vi "AES-InvCipher-text.vi"(5 "Initializer Vector":string, 7 "Operation Mode":T1, 8 "error in (no error)":errorcluster, 9 "inv-cipher [U8]":u8[](array[numeric]), 10 "Cipher Key":string, 11 "ciphertext":string) -> (0 "error out":errorcluster, 1 "inv-cipher out":u8[](array[numeric]), 3 "plaintext":string)   [LabVIEW 2020, in "Encryption.lvlib"]
doc: "Decipher a AES-encrypted message using the Cipher key and Operation Mode.\n\nCAUTION:\nThis VI is not secure, it does not protect the memory of the encryption, key and unencrypted data.\n\n(c) Ton Plomp, 2011\nTHIS SOFTWARE IS PROVIDED AS IS, AND ANY WARRANTY IS REJECTED"
uses:
  Encryption.lvlib
  AES-Modes.ctl
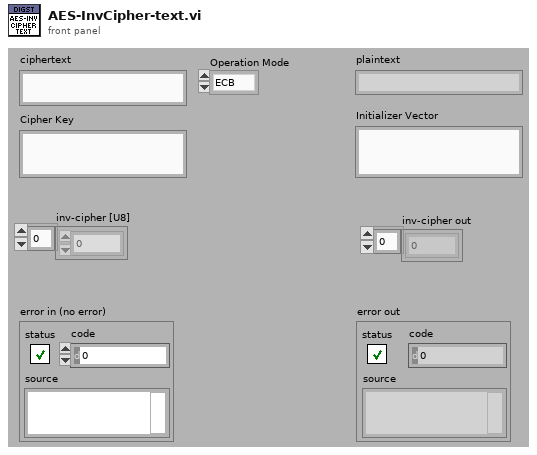
[diagram p1: front panel]
types:
  T1 = typedef "Encryption.lvlib/AES-Modes.ctl" = enum16{"ECB", "CBC", "CFB128", "OFB"}
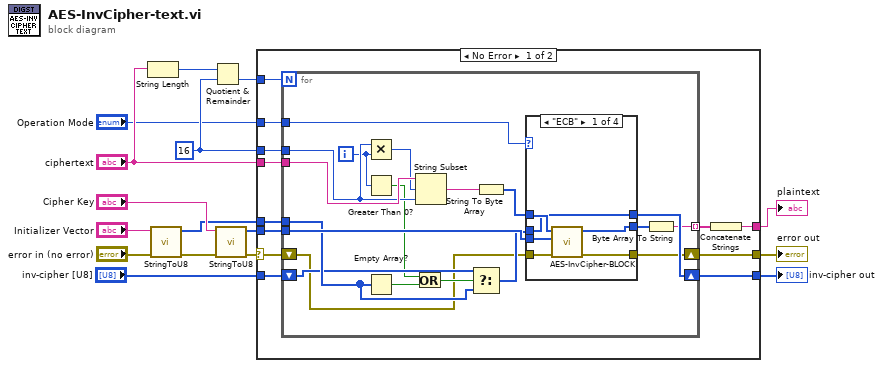
[diagram p0: block diagram]
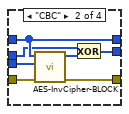
[diagram p2: hidden frame]
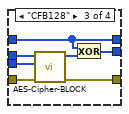
[diagram p3: hidden frame]
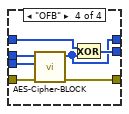
[diagram p4: hidden frame]
diagram:
  w9 = 16 ("y")
  n1 = String Length(string="ciphertext") -> (length=w13:i32)
  n2 = call "StringToU8.vi"("error in (no error)"="error in (no error)", "HEX text in"="Initializer Vector") -> ("error out"=w6:errorcluster, "ArrayU8 out"=w4:u8[])  [unwired: 8 in]
  n3 = Quotient & Remainder(x=w13, y=w9) -> (floor(x/y)=w8:i32)  [unwired: 1 out]
  n4 = call "StringToU8.vi"("error in (no error)"=w6, "HEX text in"="Cipher Key") -> ("error out"=w12:errorcluster, "ArrayU8 out"=w11:u8[])  [unwired: 8 in]
  n5 = case shown="No Error" w12 {
    selector: w12 -> [w24 w76]
    tunnel: "ciphertext" -> [w28 _]
    tunnel: [w23 w76] -> w15
    tunnel: w11 -> [w27 _]
    tunnel: w8 -> [w26 _]
    tunnel: w9 -> [w25 _]
    tunnel: [w21 _] -> w10
    tunnel: w4 -> [w19 _]
    tunnel: "Operation Mode" -> [w20 _]
    tunnel: "inv-cipher [U8]" -> [w18 w75]
    tunnel: [w17 w75] -> w1
    frame No Error {
      n6 = for {
        N: w26 -> [_]
        tunnel: w28 -> [w46]
        tunnel: w27 -> [w47]
        tunnel: w25 -> [w44]
        shift-right: [w39] -> w23
        shift-left: w24 -> [w31]
        tunnel: [w41] -> w22 mode=indexing
        shift-right: [w42] -> w17
        shift-left: w18 -> [w37]
        tunnel: w20 -> [w43]
        tunnel: w19 -> [w38]
        i -> [w35]
        n7 = Multiply(x=w44, y=w35) -> (x*y=w45:i32)
        n8 = Greater Than 0?(x=w35) -> (x > 0?=w34:bool)
        n9 = Empty Array?(array=w38) -> (empty?=w33:bool)
        n10 = Or(x=w34, y=w33) -> (x .or. y?=w32:bool)
        n11 = String Subset(string=w46, offset (0)=w45, length (rest)=w44) -> (substring=w30:string)
        n12 = Select(t=w37, s=w32, f=w38) -> (s? t:f=w36:u8[])
        n13 = String To Byte Array(string=w30) -> (unsigned byte array=w29:u8[])
        n14 = case shown="\"ECB\"" w43 {
          tunnel: w47 -> [w53 w60 w67 w74]
          tunnel: w29 -> [w52 w57 w61 w69]
          tunnel: w31 -> [w51 w59 w66 w73]
          tunnel: [w50 w54 w63 w71] -> w40
          tunnel: [w49 w58 w65 w72] -> w39
          tunnel: w36 -> [w48 w56 w62 w70]
          tunnel: [w48 w57 w61 w68] -> w42
          frame "ECB" {
            n15 = call "AES-InvCipher-BLOCK.vi"("error in (no error)"=w51, "Cipher Key"=w53, "cipher [U8]"=w52) -> ("error out"=w49:errorcluster, "plain [U8]"=w50:u8[])  [unwired: 7 in]
          }
          frame "CBC" {
            n16 = call "AES-InvCipher-BLOCK.vi"("error in (no error)"=w59, "Cipher Key"=w60, "cipher [U8]"=w57) -> ("error out"=w58:errorcluster, "plain [U8]"=w55:u8[])  [unwired: 7 in]
            n17 = Exclusive Or(1:w55, 2:w56) -> (0:w54:u8[])
          }
          frame "CFB128" {
            n18 = call "AES-Cipher-BLOCK.vi"("error in (no error)"=w66, "Cipher Key"=w67, "Plain [U8]"=w62) -> ("error out"=w65:errorcluster, "cipher [U8]"=w64:u8[])  [unwired: 7 in]
            n19 = Exclusive Or(1:w64, 2:w61) -> (0:w63:u8[])
          }
          frame "OFB" {
            n20 = call "AES-Cipher-BLOCK.vi"("error in (no error)"=w73, "Cipher Key"=w74, "Plain [U8]"=w70) -> ("error out"=w72:errorcluster, "cipher [U8]"=w68:u8[])  [unwired: 7 in]
            n21 = Exclusive Or(1:w68, 2:w69) -> (0:w71:u8[])
          }
        }
        n22 = Byte Array To String(unsigned byte array=w40) -> (string=w41:string)
      }
      n23 = Concatenate Strings(w22) -> (w21:string)
    }
    frame Error {
    }
  }
  "error out" <- w15
  "plaintext" <- w10
  "inv-cipher out" <- w1
